vi "Write Return Microgrid State Msg.vi"(10 "Return Microgrid State Msg":refnum<class "Return Microgrid State Msg.lvclass">, 11 "SCADA in":refnum<class "EMS.lvclass">) -> (3 "SCADA out":refnum<class "EMS.lvclass">)   [LabVIEW 2018, in "EMS Core.lvlib" / "EMS.lvclass"]
uses:
  EMS.lvclass
  EMS Messages/Return Microgrid State Msg/Return Microgrid State Msg.lvclass
  EMS.lvclass/EMS.ctl
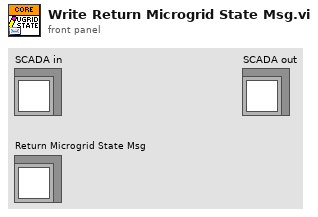
[diagram p1: front panel]
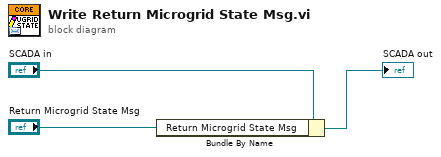
[diagram p0: block diagram]
diagram:
  n1 = Bundle By Name(cluster="SCADA in", "Return Microgrid State Msg"="Return Microgrid State Msg") -> (→"SCADA out":refnum<class "EMS.lvclass">)
